vi "Initialize.vi"(6 "Reset (True)":bool=TRUE, 7 "Serial Configuration":T1={"Baud Rate"=9600, "Parity"=0, "Data Bits"=7, "Stop Bits"=10, "Flow Control"=0} {"Flow Control" items=["None", "XON/XOFF", "RTS/CTS", "XON/XOFF & RTS/CTS", "DTR/DSR", "XON/XOFF & DTR/DSR"]; "Stop Bits" items=["1.0"=10, "1.5"=15, "2.0"=20]; "Data Bits" items=["7"=7, "8"=8]; "Parity" items=["None", "Odd", "Even", "Mark", "Space"]; "Baud Rate" items=["300"=300, "600"=600, "1200"=1200, "2400"=2400, "4800"=4800, "9600"=9600, "19200"=19200]}, 8 "error in (no error)":errorcluster, 9 "Error Query (False)":bool, 10 "ID Query (True)":bool=TRUE, 11 "VISA resource name":refnum<visa-resource-name>) -> (0 "error out":errorcluster, 3 "VISA resource name out":refnum<visa-resource-name>)   [LabVIEW 2012, in "Keithley 2600 Series.lvlib"]
doc: "Establishes communication with the instrument and optionally performs an instrument identification query and/or an instrument reset. It also places the instrument in a default state needed for other instrument driver operations. Therefore, call this VI before calling other instrument driver VIs for this instrument. Generally, you need to call the Initialize VI only once at the beginning of an application."
uses:
  Keithley 2600 Series.lvlib
  Private/GlobalVariables.vi
panel:
  # "(c) 2008 Keithley Instruments, Inc.  ALL RIGHTS RESERVED."
  # "Automatic"
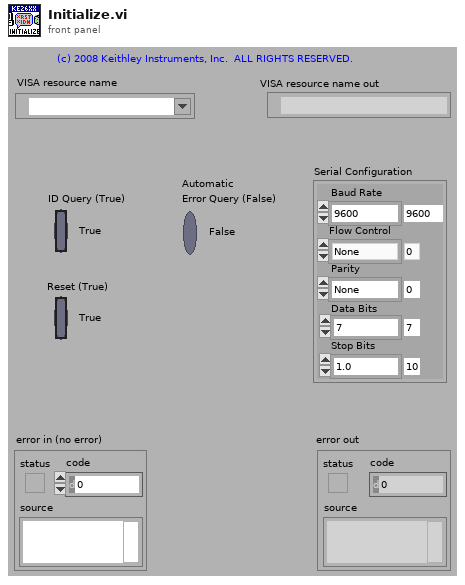
[diagram p1: front panel]
types:
  T1 = cluster{"Baud Rate":u32, "Parity":u16, "Data Bits":u16, "Stop Bits":u16, "Flow Control":u16}
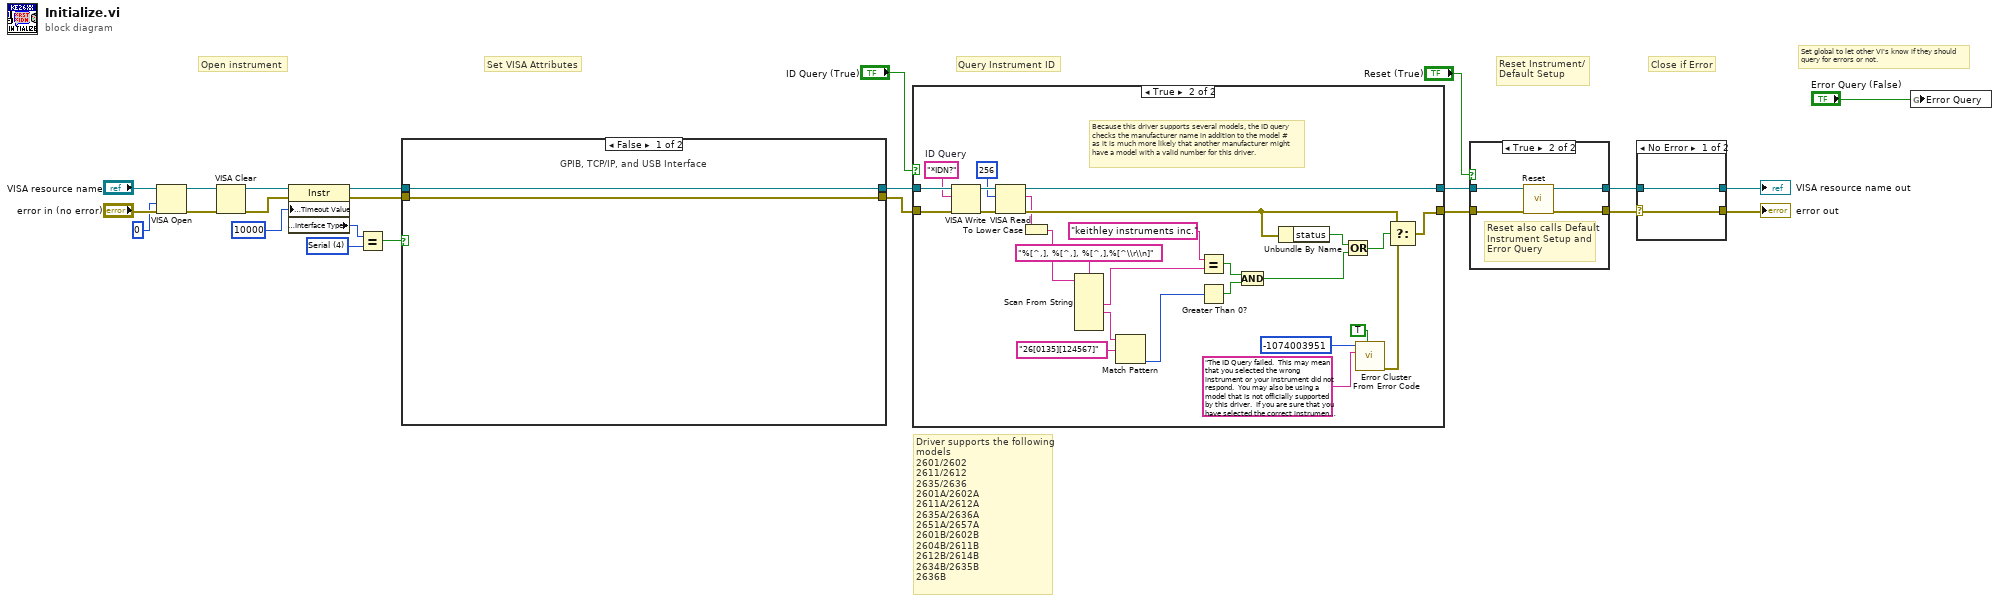
[diagram p0: block diagram]
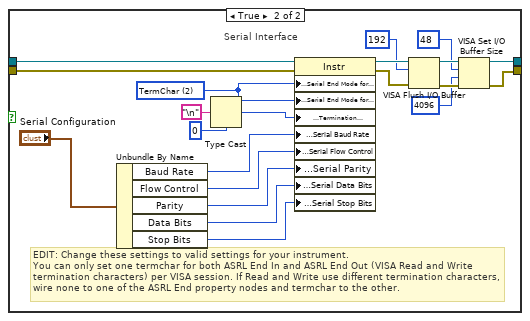
[diagram p2: hidden frame]
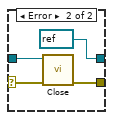
[diagram p3: hidden frame]
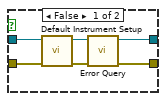
[diagram p4: hidden frame]
diagram:
  w11 = u16 4 items=["GPIB"=1, "VXI"=2, "GPIB-VXI"=3, "Serial"=4, "PXI"=5, "TCPIP"=6, "USB"=7] ("Interface Information:Interface Type")
  # "Driver supports the following models\n2601/2602\n2611/2612\n2635/2636\n2601A/2602A\n2611A/2612A\n2635A/2636A\n2651A/2657A\n2601B/2602B\n2604B/2611B\n2612B/2614B\n2634B/2635B\n2636B"
  # "Set global to let other VI's know if they should\nquery for errors or not."
  # "Set VISA Attributes"
  # "Close if Error"
  # "Query Instrument ID"
  # "Reset Instrument/\nDefault Setup"
  # "Open instrument"
  n1 = VISA Open(access mode=u32 0, error in (no error)="error in (no error)", VISA resource name="VISA resource name") -> (VISA resource name=w9:refnum<visa-resource-name>, error out=w8:errorcluster)  [unwired: 2 out]
  n2 = VISA Clear(VISA resource name=w9, error in (no error)=w8) -> (VISA resource name out=w7:refnum<visa-resource-name>, error out=w6:errorcluster)
  n3 = property class="Instr"(reference=w7, error in=w6, "General Settings:Timeout Value"=u32 10000) -> (reference out=w14:refnum<visa-resource-name>, error out=w13:errorcluster, "Interface Information:Interface Type"=w18:u16)
  n4 = Equal?(x=w18, y=w11) -> (x = y?=w12:bool)
  n5 = case shown="False" w12 {
    tunnel: [w25 w44] -> w16
    tunnel: [w26 w41] -> w15
    tunnel: w14 -> [w25 w46]
    tunnel: w13 -> [w26 w47]
    frame False {
      # "GPIB, TCP/IP, and USB Interface"
    }
    frame True {
      w34 = u16 2 items=["None", "LastBit", "TermChar"] ("Serial Settings:Serial End Mode for Reads")
      # "EDIT: Change these settings to valid settings for your instrument.\nYou can only set one termchar for both ASRL End In and ASRL End Out (VISA Read and Write termination characters) per VISA session. If Read and Write use different termination characters, wire none to one of the ASRL End property nodes and termchar to the other."
      # "Serial Interface"
      n6 = Unbundle By Name("Serial Configuration") -> ("Baud Rate"=w32:u32, "Flow Control"=w28:u16, "Parity"=w30:u16, "Data Bits"=w31:u16, "Stop Bits"=w27:u16)
      n7 = Type Cast(type=u8 0, x="\n" ("Line Feed Constant")) -> (*(type *) &x=w33:u8)
      n8 = property class="Instr"(reference=w46, error in=w47, "Serial Settings:Serial End Mode for Reads"=w34, "Serial Settings:Serial End Mode for Writes"=w34, "Message Based Settings:Termination Character"=w33, "Serial Settings:Serial Baud Rate"=w32, "Serial Settings:Serial Flow Control"=w28, "Serial Settings:Serial Parity"=w30, "Serial Settings:Serial Data Bits"=w31, "Serial Settings:Serial Stop Bits"=w27) -> (reference out=w40:refnum<visa-resource-name>, error out=w43:errorcluster)
      n9 = VISA Flush I/O Buffer(VISA resource name=w40, mask (16)=u16 192, error in (no error)=w43) -> (VISA resource name out=w45:refnum<visa-resource-name>, error out=w42:errorcluster)
      n10 = VISA Set I/O Buffer Size(VISA resource name=w45, mask (16)=u16 48, size (4096)=u32 4096 ("size (0)"), error in (no error)=w42) -> (VISA resource name out=w44:refnum<visa-resource-name>, error out=w41:errorcluster)
    }
  }
  n11 = case shown="True" "ID Query (True)" {
    tunnel: [w48 w75] -> w23
    tunnel: [w49 w72] -> w24
    tunnel: w16 -> [w49 w73]
    tunnel: w15 -> [w48 w74]
    frame False {
    }
    frame True {
      w68 = "*IDN?"  # ID Query
      # "Because this driver supports several models, the ID query\nchecks the manufacturer name in addition to the model #\nas it is much more likely that another manufacturer might\nhave a model with a valid number for this driver."
      n12 = VISA Write(VISA resource name=w73, write buffer=w68, error in (no error)=w74) -> (VISA resource name out=w71:refnum<visa-resource-name>, error out=w70:errorcluster)  [unwired: 1 out]
      n13 = VISA Read(VISA resource name=w71, byte count=u32 256, error in (no error)=w70) -> (VISA resource name out=w72:refnum<visa-resource-name>, read buffer=w60:string, error out=w63:errorcluster)  [unwired: 1 out]
      n14 = To Lower Case(string=w60) -> (all lower case string=w54:string)
      n15 = Scan From String(format string="%[^,], %[^,], %[^,],%[^\\r\\n]", input string=w54) -> (output 1=w52:string, output 2=w50:string)  [unwired: 4 in, 7 out]
      n16 = Match Pattern(string=w50, regular expression="26[0135][124567]") -> (offset past match=w58:i32)  [unwired: 4 out]
      n17 = Equal?(x="keithley instruments inc." ("regular expression"), y=w52) -> (x = y?=w51:bool)
      n18 = Greater Than 0?(x=w58) -> (x > 0?=w57:bool)
      n19 = And(x=w51, y=w57) -> (x .and. y?=w56:bool)
      n20 = Unbundle By Name(w63) -> ("status"=w62:bool)
      n21 = Or(x=w62, y=w56) -> (x .or. y?=w61:bool)
      n22 = call <vilib>:"Error Cluster From Error Code.vi"("show call chain? (False)"=TRUE, "error message (\"\")"="The ID Query failed.  This may mean that you selected the wrong instrument or your instrument did not respond.  You may also be using a model that is not officially supported by this driver.  If you are sure that you have selected the correct instrument and it is responding, try disabling the ID Query." ("Source (VI Name)"), "error code (0)"=-1074003951 ("Code")) -> ("error out"=w67:errorcluster)  [unwired: 1 in, 5 out]
      n23 = Select(t=w63, s=w61, f=w67) -> (s? t:f=w75:errorcluster)
    }
  }
  n24 = case shown="True" "Reset (True)" {
    tunnel: w23 -> [w80 w82]
    tunnel: [w77 w85] -> w2
    tunnel: w24 -> [w81 w83]
    tunnel: [w78 w84] -> w3
    frame False {
      n25 = call "Default Instrument Setup.vi"("error in (no error)"=w80, "VISA resource name"=w81) -> ("error out"=w76:errorcluster, "VISA resource name out"=w79:refnum<visa-resource-name>)  [unwired: 8 out]
      n26 = call "Error Query.vi"("error in (no error)"=w76, "VISA resource name"=w79) -> ("error out"=w77:errorcluster, "VISA resource name out"=w78:refnum<visa-resource-name>)  [unwired: 8 out]
    }
    frame True {
      # "Reset also calls Default Instrument Setup and Error Query"
      n27 = call "Reset.vi"("error in (no error)"=w82, "VISA resource name"=w83) -> ("error out"=w85:errorcluster, "VISA resource name out"=w84:refnum<visa-resource-name>)  [unwired: 8 out]
    }
  }
  n28 = case shown="No Error" w2 {
    selector: w2 -> [w86 w89]
    tunnel: w3 -> [w87 w90]
    tunnel: [w87 refnum<visa-resource-name> refnum ("VISA resource name out")] -> w5
    tunnel: [w86 w91] -> w4
    frame No Error {
    }
    frame Error {
      n29 = call "Close.vi"("error in (no error)"=w89, "VISA resource name"=w90) -> ("error out"=w91:errorcluster)  [unwired: 9 out]
    }
  }
  "VISA resource name out" <- w5
  "error out" <- w4
  n30 = global write "GlobalVariables.vi" "Error Query"("Error Query (False)") -> ()
